vi "Untitled 8.vi"() -> ()   [LabVIEW 2017]
panel:
  in  "Tab Control 4":T1(tab)
  in  "nm --> cm-1":bool
  out "?":string
  in  "Dim X":dbl=40.0
  in  "Dim Y":dbl=40.0
  out "Data Numeric":dbl
  in  "P1 start (nm/cm-1)":dbl=520.0
  in  "P1 end (nm/cm-1)":dbl=750.0
  in  "Graph save start":i32
  in  "Graph save end":i32=1600
  in  "Remove background?":bool
  in  "Save Data? 2":bool
  in  "Find peak?":bool
  in  "Gaussian fit?":bool
  out "best fit parameters":dbl[][](array[numeric])
  out "Peaks intensity":dbl[][](array[numeric])
  out "How many peak find":i32[](array[numeric])
  out "Biggest intensity":dbl[](array[numeric])
  in  "Start in Xth spectrum":i32=1
  in  "Average how many data":i32=10
  in  "Save Data?":bool
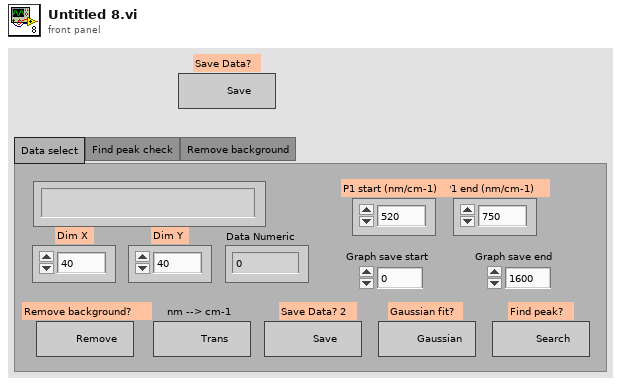
[diagram p1: front panel]
types:
  T1 = enum32{"Data select", "Find peak check", "Remove background"}
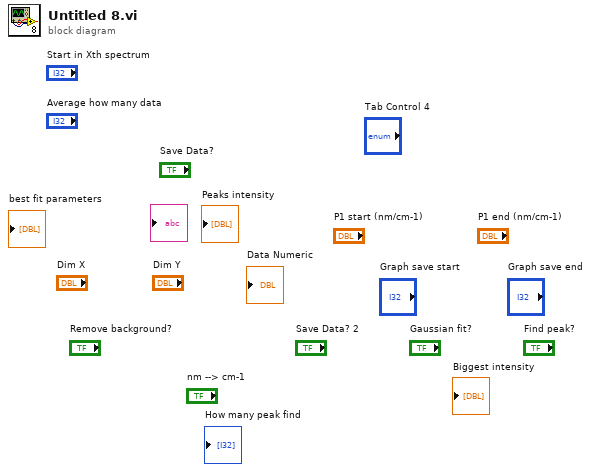
[diagram p0: block diagram]
diagram:
